vi "Insert Value (Boolean).vi"(7 "key":string, 8 "error in (no error)":errorcluster, 10 "value":bool, 11 "JSON Value in":refnum<class "JSON Value.lvclass">) -> (0 "error out":errorcluster, 1 "replaced":bool, 3 "JSON Value out":refnum<class "JSON Value.lvclass">)   [LabVIEW 2016, in "JSON Value.lvclass"]
uses:
  JSON Value.lvclass
  New JSON Value/New JSON (Boolean).vi
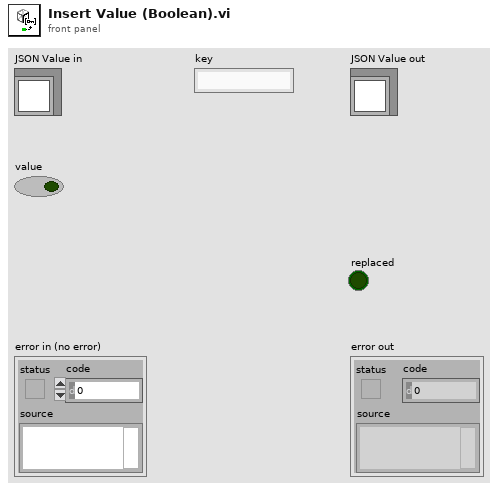
[diagram p1: front panel]
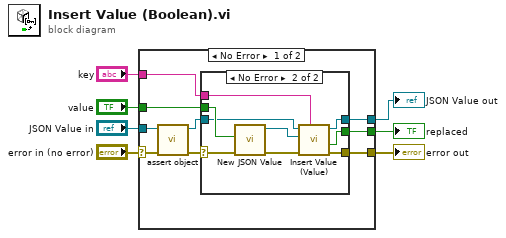
[diagram p0: block diagram]
diagram:
  n1 = case shown="No Error" "error in (no error)" {
    selector: "error in (no error)" -> [w11 w29]
    tunnel: [w13 w29] -> w5
    tunnel: [w16 w28] -> w7
    tunnel: "JSON Value in" -> [w9 w28]
    tunnel: "key" -> [w15 _]
    tunnel: "value" -> [w14 _]
    tunnel: [w12 _] -> w6
    frame No Error {
      n2 = call "assert object.vi"("error in (no error)"=w11, "JSON Value in"=w9) -> ("error out"=w10:errorcluster, "JSON Value out"=w8:refnum<class "JSON Value.lvclass">)  [unwired: 8 in]
      n3 = case shown="No Error" w10 {
        selector: w10 -> [w17 w26]
        tunnel: [w18 w24] -> w16
        tunnel: w15 -> [_ w20]
        tunnel: w14 -> [_ w27]
        tunnel: [w17 w21] -> w13
        tunnel: [_ w23] -> w12
        tunnel: w8 -> [w18 w25]
        frame Error {
        }
        frame No Error {
          n4 = call-poly "New JSON Value.vi"("error in (no error)"=w26, "value"=w27) -> ("error out"=w22:errorcluster, "JSON Value out"=w19:refnum<class "JSON Value.lvclass">)  [unwired: 8 in]
          n5 = call "Insert Value (Value).vi"("key"=w20, "error in (no error)"=w22, 10:"JSON Value in"=w19, 11:"JSON Value in"=w25) -> ("error out"=w21:errorcluster, "replaced"=w23:bool, "JSON Value out"=w24:refnum<class "JSON Value.lvclass">)  [unwired: 5 in]
        }
      }
    }
    frame Error {
    }
  }
  "error out" <- w5
  "JSON Value out" <- w7
  "replaced" <- w6
